vi "ESP_RT_UDP_read_and_trigger.vi"(7 "Data_In":dbl[](array[numeric]), 8 "error in":errorcluster, 9 "UDP_read_timeout(ms)":i32, 10 "Trigger_task_in":refnum<k21>, 11 "connection ID":refnum<k16>) -> (0 "error out":errorcluster, 1 "ESP_Data(1x64)":dbl[][](array[numeric]), 2 "Trigger_task_out":refnum<k21>, 3 "connection ID out":refnum<k16>, 4 "ESP_Index_Data":dbl[](array[numeric]), 6 "UDP_status":string)   [LabVIEW 2021]
uses:
  <vilib>/DAQmx/write.llb/DAQmx Write (Digital Bool 1Line 1Point).vi
  <vilib>/DAQmx/miscellaneous.llb/DAQmx Fill In Error Info.vi
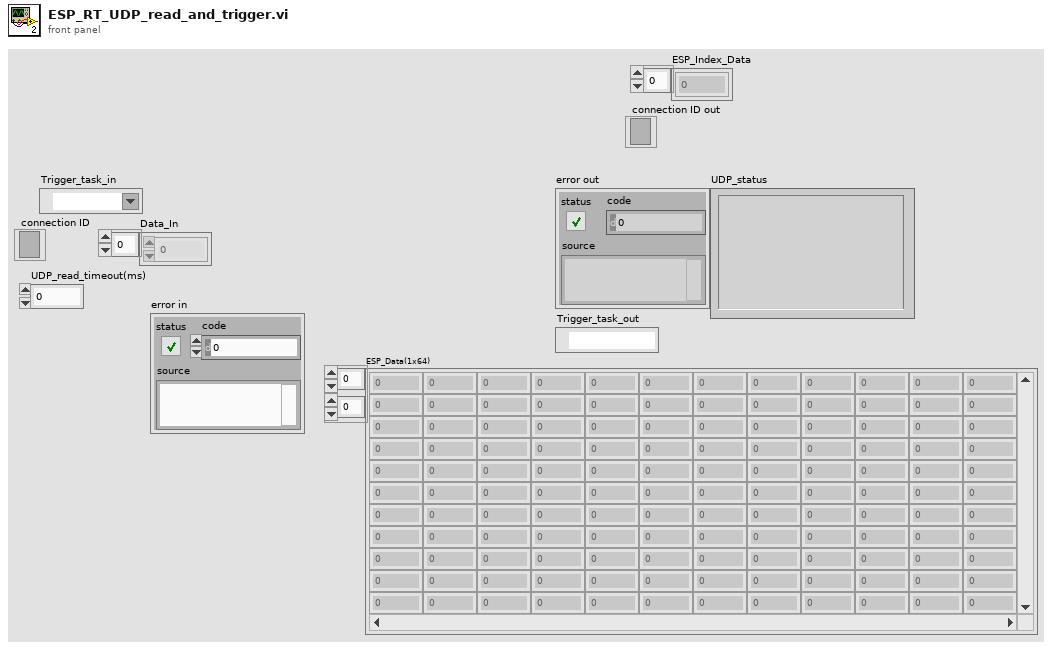
[diagram p1: front panel]
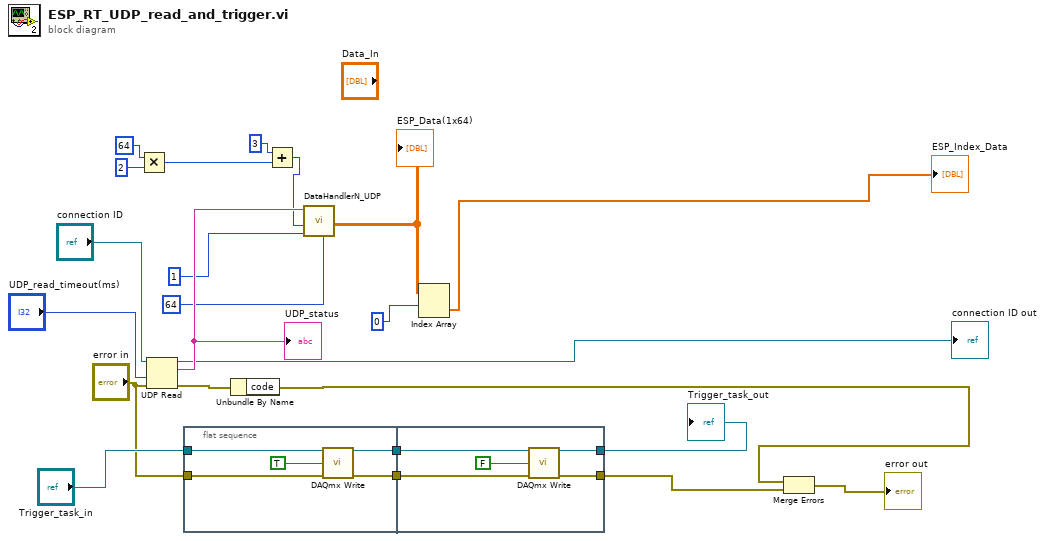
[diagram p0: block diagram]
diagram:
  n1 = Multiply(x=64, y=2) -> (x*y=w4:i32)
  n2 = UDP Read(connection ID="connection ID", timeout ms (25000)="UDP_read_timeout(ms)", 8:"error in") -> (data out=w18:string, error out=w11:errorcluster, 3:→"connection ID out":refnum<k16>)  [unwired: 1 in, 2 out]
  "UDP_status" <- w18
  n3 = flat-sequence {
    tunnel: "error in" -> [w27]
    tunnel: "Trigger_task_in" -> [w26]
    tunnel: [w25] -> w22
    tunnel: [w24] -> w21
    tunnel: [w30] -> w20
    tunnel: [w31] -> w12
    tunnel: w22 -> [w32]
    tunnel: w21 -> [w29]
    frame #0 {
      n4 = call-poly <vilib>:"DAQmx Write.vi"("task/channels in"=w26, "data"=TRUE, "error in"=w27) -> ("task out"=w24:refnum<k21>, "error out"=w25:errorcluster)  [unwired: 10 in, 1 out]
    }
    frame #1 {
      n5 = call-poly <vilib>:"DAQmx Write.vi"("task/channels in"=w29, "data"=FALSE, "error in"=w32) -> ("task out"=w30:refnum<k21>, "error out"=w31:errorcluster)  [unwired: 10 in, 1 out]
    }
  }
  n6 = Unbundle By Name(w11) -> ()  [unwired: 1 out]
  n7 = Add(x=3, y=w4) -> (x+y=w1:i32)
  n8 = call "DataHandlerN_UDP.vi"("Data Cycles Per Buffer"=1, "Rx Packet Byte size"=w1, "data out"=w18, "Nchan"=64) -> ("Data"=w13:dbl[][])  [unwired: 2 in, 3 out]
  "ESP_Data(1x64)" <- w13
  n9 = Index Array(array=w13, index (row)=0 ("Data Cycles Per Buffer")) -> (element=→"ESP_Index_Data":dbl[])  [unwired: 1 in]
  n10 = Merge Errors(w11, w12) -> (→"error out":errorcluster)
  "Trigger_task_out" <- w20
